vi "Text control 1 v0.2.vi"() -> ()   [LabVIEW 2016]
panel:
  in  "Panel Controls 2":T1={"Emergency Stop"=refnum, "TransGraph Max"=1e-05, "Text/Graph (text=false)"=TRUE, "TransGraph Min"=1e-11} {"TransGraph Min" format="%.2e"; "TransGraph Max" format="%.2e"}
  out "Currently running:":string="#output s 0 0 0 -0.008 0.008 0.002"
  in  "Lines left to run:":string
  in  "Standby":T2
  in  "Full Reset":bool
  in  "SMU4":cluster{"on/off":bool, "Voltage":dbl} {"Voltage" min=-100.0 max=100.0 format="%.2f"}
  in  "Source/Drain\nRange":u8(slide)=6 max=11 scale=0.0..11.0
  in  "Source/Drain\nRange mode":u16(ring) items=["Auto", "Limited", "Fixed"]
  in  "Gate Range":u8(slide)=6 max=11 scale=0.0..11.0
  in  "Gate Range\nmode":u16(ring) items=["Auto", "Limited", "Fixed"]
  in  "Gate":T3={"Gate Start"=0.0, "Gate Stop"=2.0, "Gate Step (linear only)"=1.0, "Gate Compliance"=0.0001, "Gate PComp"=0.0, "Range mode"=0, "Range"=6} {"Range" max=11 scale=0.0..11.0; "Range mode" items=["Auto", "Limited", "Fixed"]; "Gate PComp" format="%^.2e"; "Gate Compliance" format="%^.2e"; "Gate Step (linear only)" format="%^.4e"; "Gate Stop" format="%^.4e"; "Gate Start" format="%^.4e"}
  in  "Drain 2":T4={"Drain Start"=0.0, "Drain Stop"=2.0, "Drain Compliance"=0.0001, "Drain Step"=1.0, "Drain PComp"=0.0, "Range mode"=0, "Range"=6} {"Range" max=11 scale=0.0..11.0; "Range mode" items=["Auto", "Limited", "Fixed"]; "Drain PComp" format="%^.2e"; "Drain Step" format="%^.4e"; "Drain Compliance" format="%^.2e"; "Drain Stop" format="%^.4e"; "Drain Start" format="%^.4e"}
  in  "Timings 2":T5={"integration time"=0, "Short/Long integration time"=0.00064, "hold time (sec)"=0.0, "delay time (sec)"=0.0, "Step Time (0 disables)"=0.0, "sweep method"=0, "Pulse period"=0.005, "Base voltage"=0.0, "Pulse width"=0.0005} {"Pulse width" min=0.0005 max=0.1 step=0.0001 format="%.4f"; "Base voltage" format="%^.4e"; "Pulse period" min=0.005 max=1.0 step=0.0001 format="%.4f"; "sweep method" items=["Continuous", "Pulsed"]; "Step Time (0 disables)" format="%.2f"; "delay time (sec)" format="%.4f"; "hold time (sec)" format="%.4f"; "Short/Long integration time" format="%^.0e"; "integration time" scale=0.0..2.0}
  in  "Panel Controls":T6={"Emergency Stop"=refnum, "TransGraph Max"=1e-05, "Text/Graph (text=false)"=TRUE} {"TransGraph Max" format="%.2e"}
  in  "Interrupt run":bool
  in  "Drain: Compliance":dbl=0.001 format="%.8f"
  in  "Gate: Compliance":dbl=0.001 format="%.8f"
  out "Path":path=path "C:/users/rlp38/09Apr2009LTtesting/test2.txt"
  in  "hold time /s":dbl format="%.2f"
  in  "delay time /s":dbl format="%.2f"
  in  "integration time":u32(slide)=1 max=2 step=1 scale=0.0..2.0
  in  "Integration time (short)":dbl=0.0019 min=8e-05 max=0.0019 step=8e-05 format="%^.0e"
  in  "Integration time (long)":dbl=0.32 min=0.04 max=2.0 step=0.02 format="%.2f"
  in  "Step delay /s":dbl format="%.2f"
  in  "Program":string="#pulsedstressV d 0.03 20 0 0.5 0.0827 5\n#\n#itime l 0.32\n#gaterangemode a\n#drainrangemode a\n#pulsed on 0.05 0 0.02\n#transfer d -10 40 1 5 40 35\n#transfer d -10 40 1 5 40 35\n#transfer d -10 40 1 5 40 35\n#output d 0 40 20 0 40 1\n#\n#\n#sample 1 0.008 221 6 0.003\n#samplei 400e-6 200 6 0.002 0.1\n#vsu2pulse -10 4\n#\n#stressV 0.016 0.03 2e-4 0.1e-3 11\n#stressI 220e-7 0.08 15\n#transfer s -1 1 0.5 -0.005 0.005 0.005\n#output s 0 0 0 -0.008 0.008 0.002\n"
  # "Syntax:\nitime [s|m|l] time(sec): [s|m|l] determines the integration time setting (small|medium|long) and time sets the value.\nNOTE: The value of the integration time has to be within the range allowed by its category (s|m|l), otherwise, the closest value will be used. (e.g. if the category is set to short but the time value is very long, the actual value used will be the maximum short integration time.\nIntegration times:\n    Short: Default: 640 us. Range: 8E-5 - 1.92E-3 seconds.\n    Medium: Fixed at 1 NPL cycle (0.02 seconds).\n    Long: Default: 16 NPL cycles (0.32 seconds). Range: 2-100 NPL cycles (0.04 seconds - 2 seconds).\ngaterangemode [a|l|f]\ndrainrangemode [a|l|f]\npulsed [on|off] PulsePeriod(sec) PulseBaseVoltage PulseONWidth(sec)\nstandby [on l off]\nwait NumMilliseconds\nwait-min NumMinutes\n# texthere = comment\ntransfer [s|d] VgStart VgStop VgStep VdStart VdStop VdStep\noutput [s|d] VgStart VgStop VgStep VdStart VdStop VdStep\nsample Vg Vd NumSamples Time(s) SampleInterval(s)\nsamplei Idg NumSamples Time(s) SampleInterval(s) VDGcompliance\n# if in doubt use SampleInterval(s) = 0.004\nstressV VG VD IGcompliance IDcompliance Duration(sec)\nstressI IDG VDGcompliance Duration(sec)\nvsu2pulse Bias Duration(s)\npulsedstressV [s|d] VEstop VgON VgOFF Period(s) PulseONwidth(s) Vd\nsample-fpp Vg Vd NumSamples Time\nresample-fpp Vg Vd\ntransfer-fpp [s|d] VgStart VgStop VgStep VdStart VdStop VdStep\noutput-fpp [s|d] VgStart VgStop VgStep VdStart VdStop VdStep"
  # "100 samples is approx 13s with medium integration"
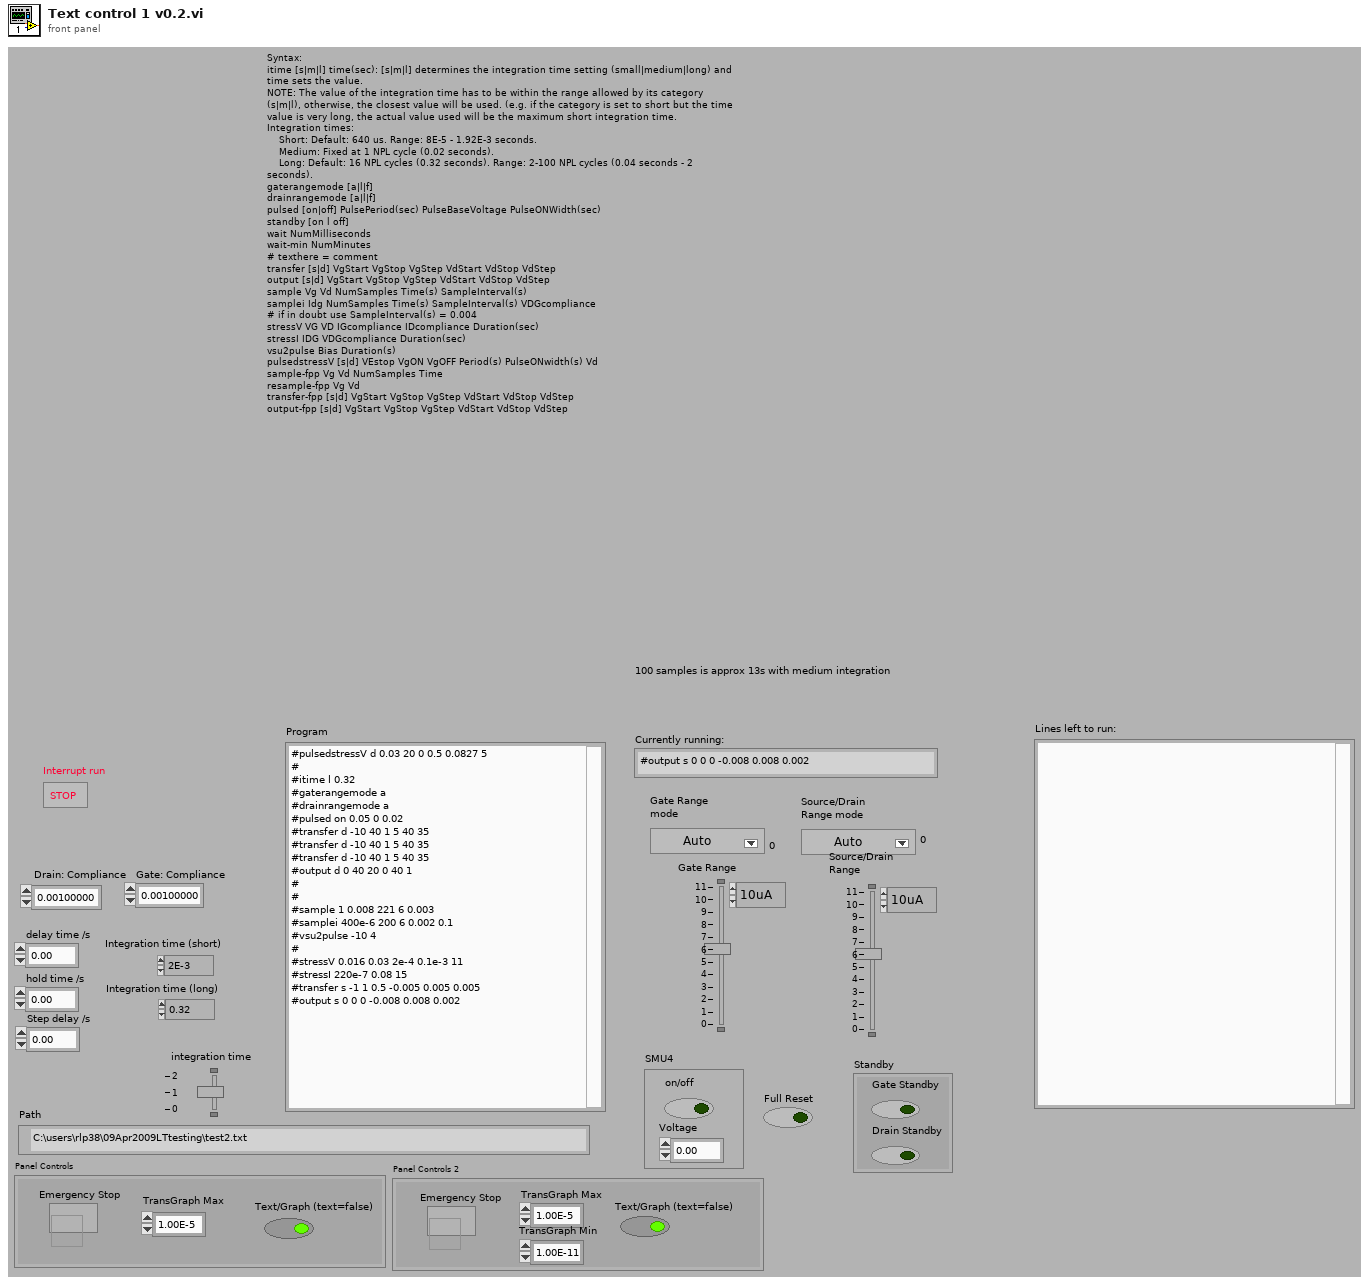
[diagram p1: front panel]
types:
  T1 = cluster{"Emergency Stop":refnum<vi>, "TransGraph Max":dbl, "Text/Graph (text=false)":bool, "TransGraph Min":dbl}
  T2 = cluster{"Gate Standby":bool, "Drain Standby":bool}
  T3 = cluster{"Gate Start":dbl, "Gate Stop":dbl, "Gate Step (linear only)":dbl, "Gate Compliance":dbl, "Gate PComp":dbl, "Range mode":u16, "Range":u8}
  T4 = cluster{"Drain Start":dbl, "Drain Stop":dbl, "Drain Compliance":dbl, "Drain Step":dbl, "Drain PComp":dbl, "Range mode":u16, "Range":u8}
  T5 = cluster{"integration time":u32, "Short/Long integration time":dbl, "hold time (sec)":dbl, "delay time (sec)":dbl, "Step Time (0 disables)":dbl, "sweep method":u16, "Pulse period":dbl, "Base voltage":dbl, "Pulse width":dbl}
  T6 = cluster{"Emergency Stop":refnum<vi>, "TransGraph Max":dbl, "Text/Graph (text=false)":bool}
  T7 = enum16{"open", "replace", "create", "open or create", "replace or create", "replace or create with confirmation"}
  T8 = cluster{"V2 Start":dbl, "V2 Step":dbl, "Number of points":i32}
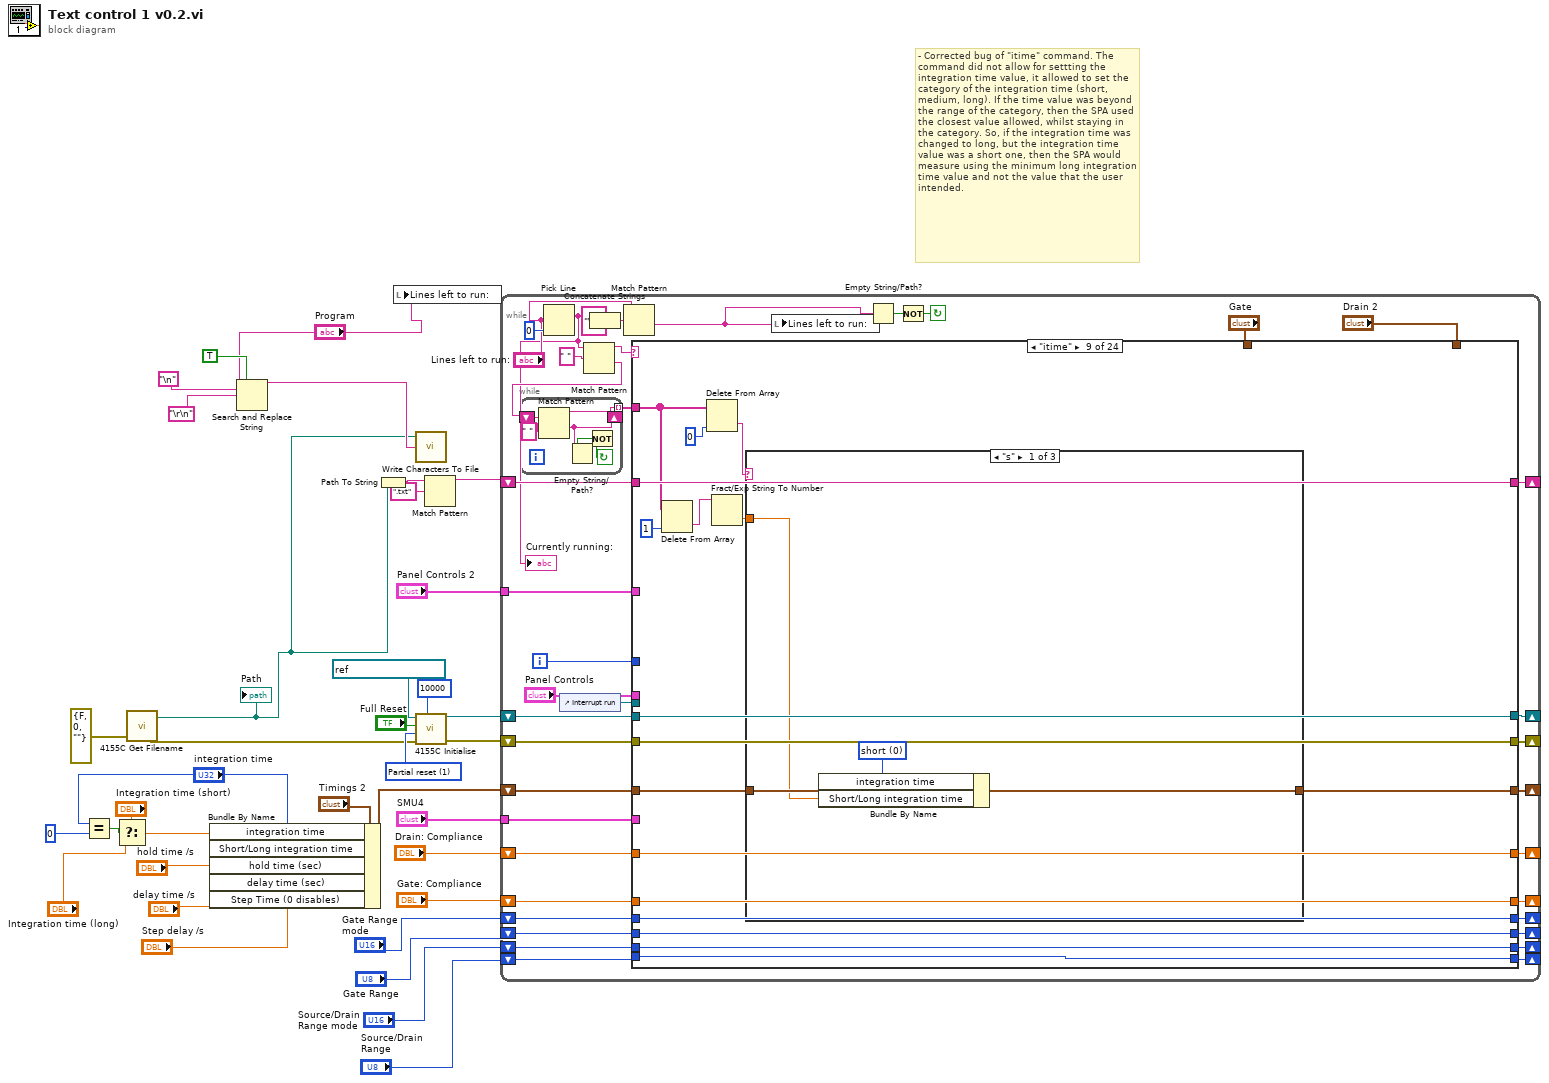
[diagram p0: block diagram]
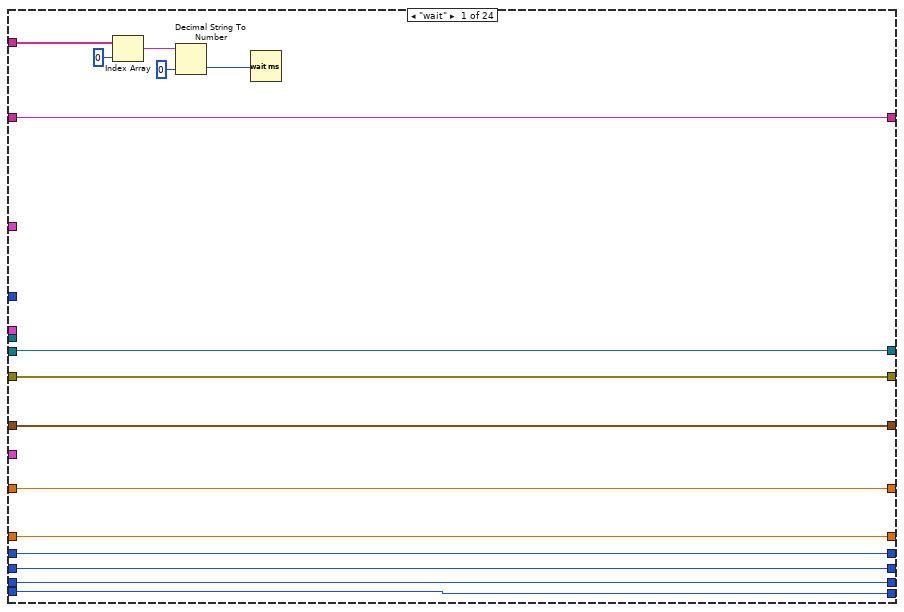
[diagram p2: hidden frame]
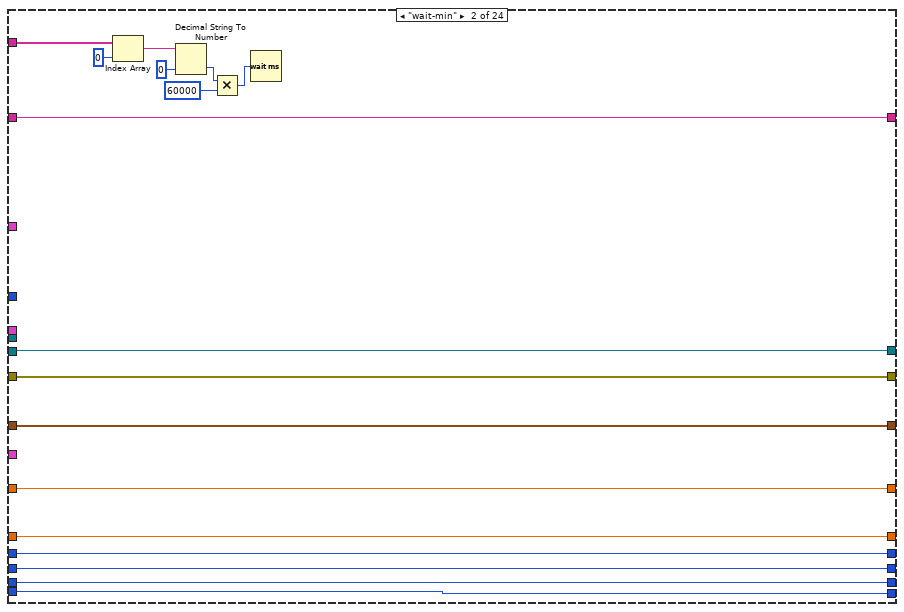
[diagram p3: hidden frame]
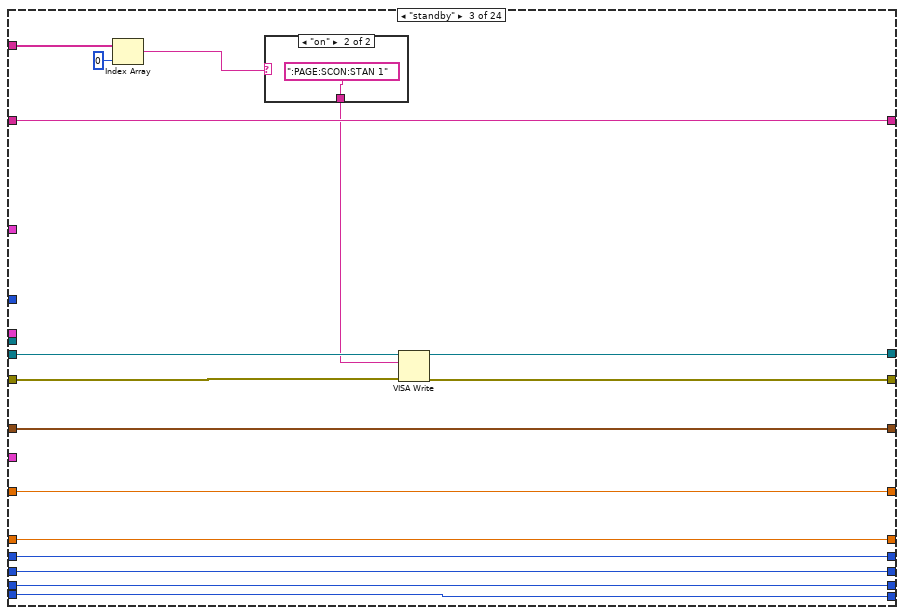
[diagram p4: hidden frame]
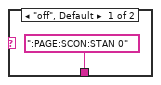
[diagram p5: hidden frame]
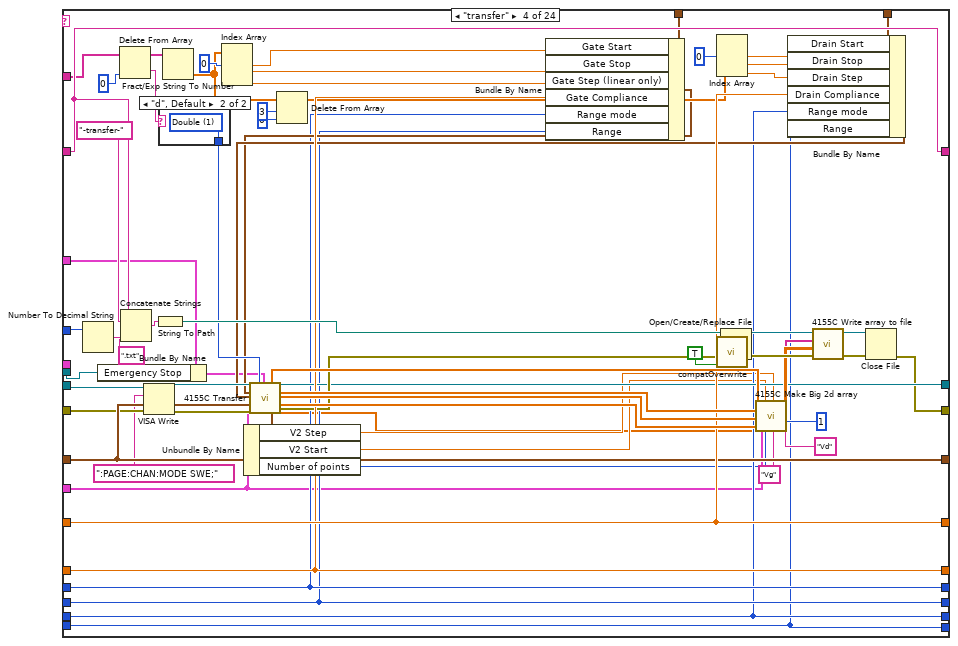
[diagram p6: hidden frame]
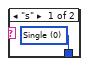
[diagram p7: hidden frame]
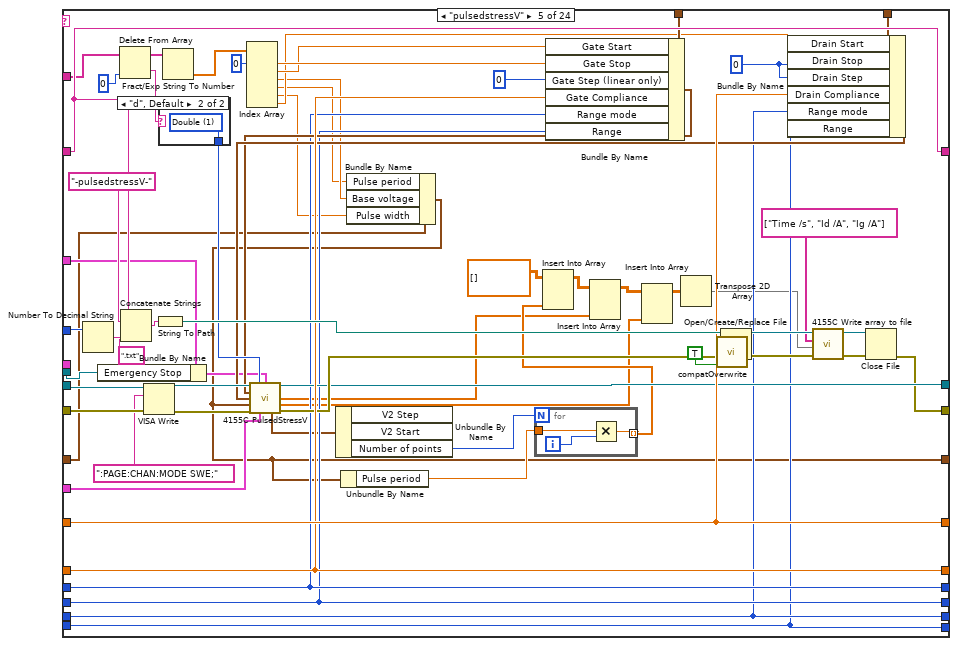
[diagram p8: hidden frame]
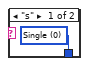
[diagram p9: hidden frame]
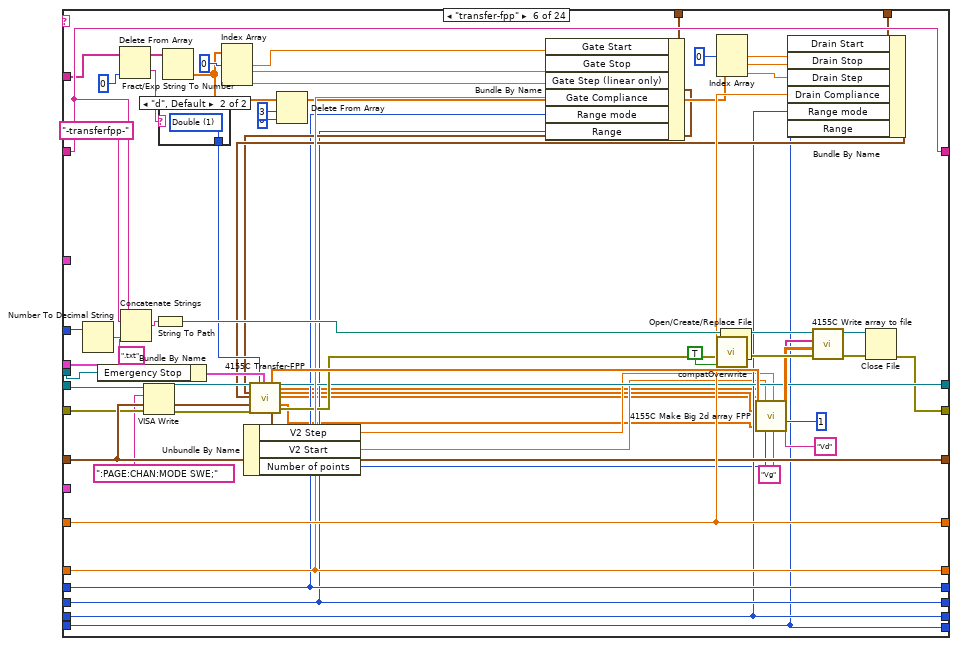
[diagram p10: hidden frame]
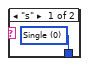
[diagram p11: hidden frame]
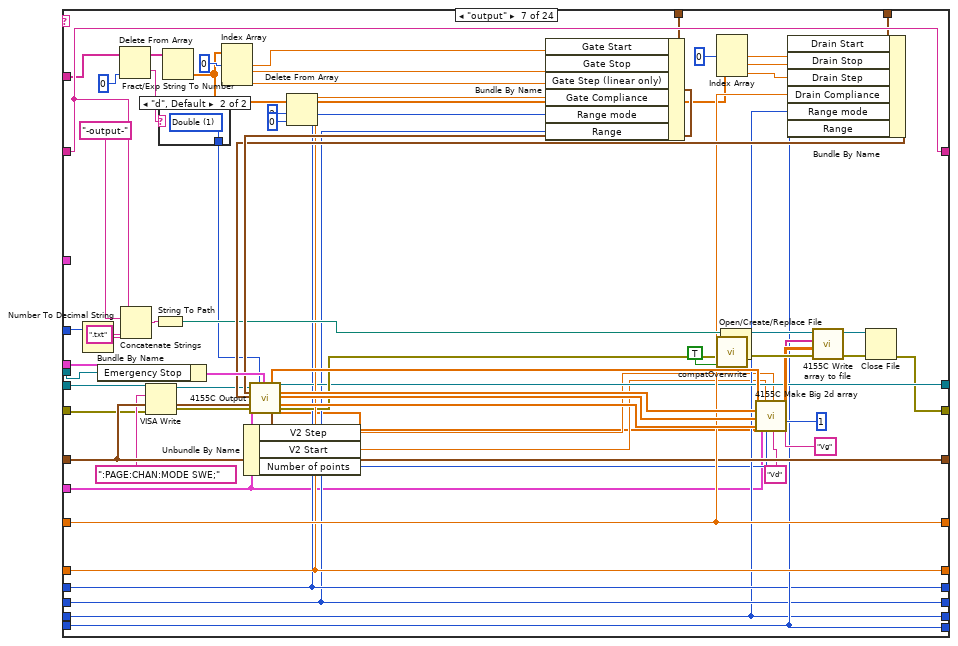
[diagram p12: hidden frame]
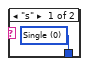
[diagram p13: hidden frame]
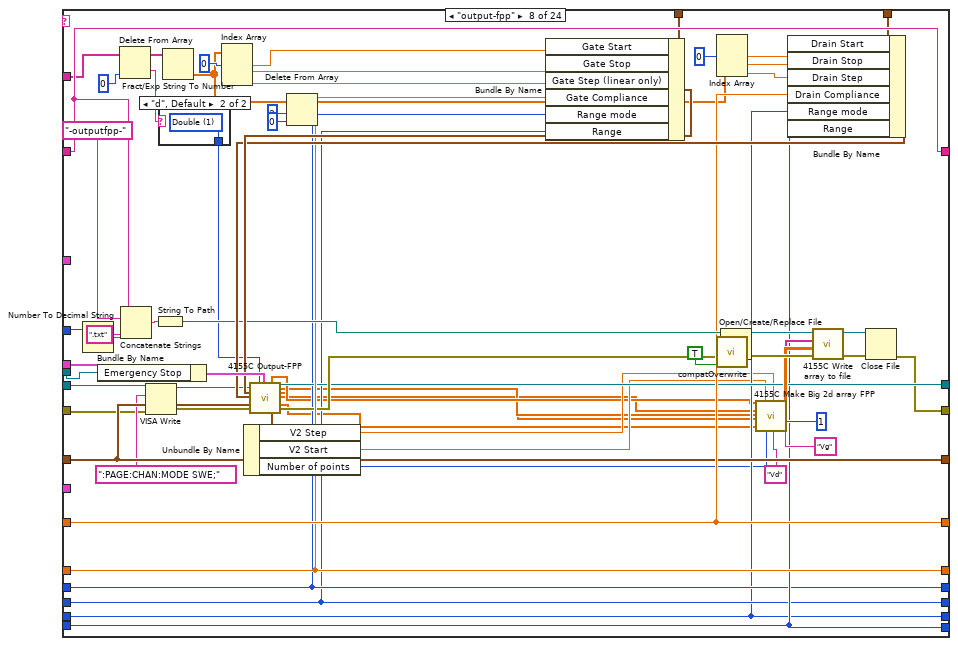
[diagram p14: hidden frame]
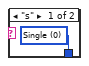
[diagram p15: hidden frame]
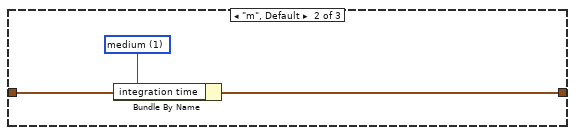
[diagram p16: hidden frame]
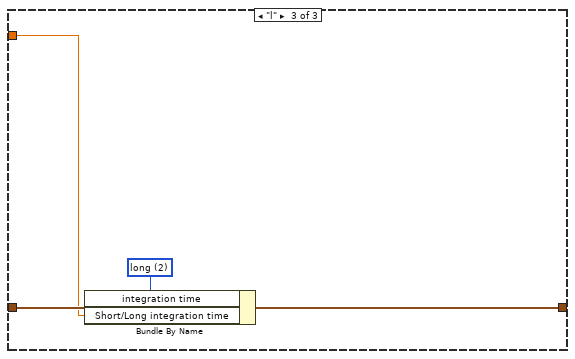
[diagram p17: hidden frame]
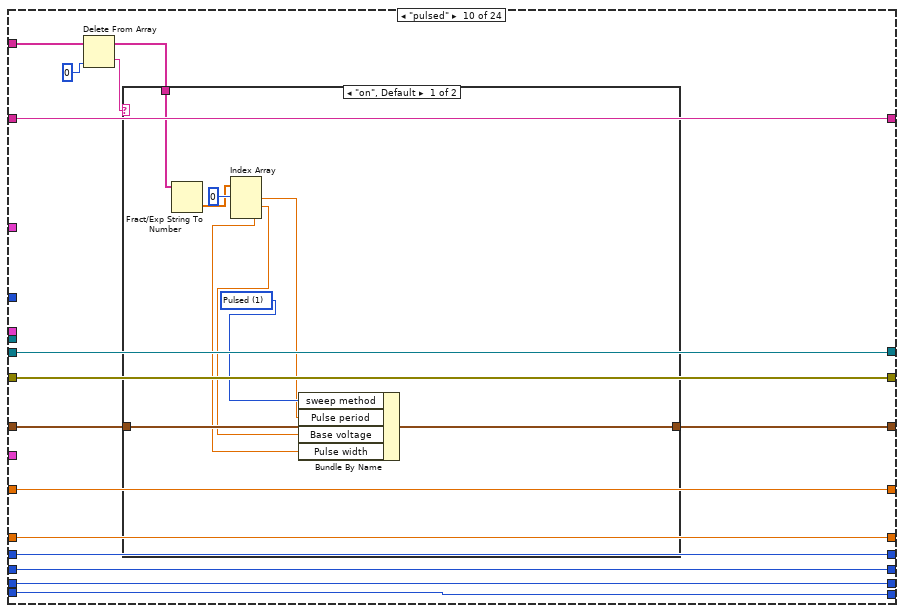
[diagram p18: hidden frame]
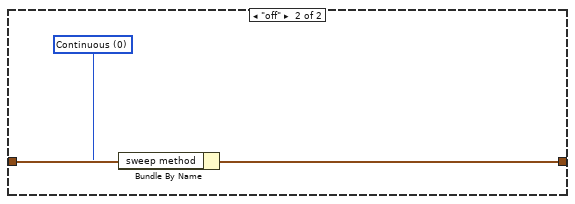
[diagram p19: hidden frame]
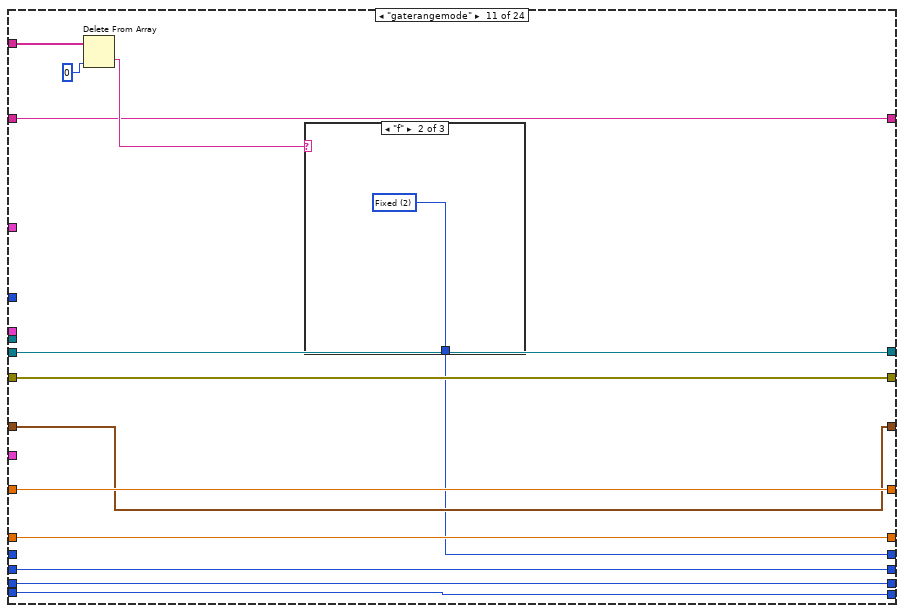
[diagram p20: hidden frame]
diagram:
  w27 = u16 1 items=["Reset All", "Partial reset"] ("Type of reset")
  # "- Corrected bug of \"itime\" command. The command did not allow for settting the integration time value, it allowed to set the category of the integration time (short, medium, long). If the time value was beyond the range of the category, then the SPA used the closest value allowed, whilst staying in the category. So, if the integration time was changed to long, but the integration time value was a short one, then the SPA would measure using the minimum long integration time value and not the value that the user intended."
  n1 = Equal?(x="integration time", y=u32 0) -> (x = y?=w31:bool)
  n2 = Select(t="Integration time (short)", s=w31, f="Integration time (long)") -> (s? t:f=w35:dbl)
  n3 = call "4155C Get Filename.vi"("error in (no error)"=errorcluster {"status"=FALSE, "code"=0, "source"=""}) -> ("error out"=w22:errorcluster, "path"=w6:path)  [unwired: 2 in, 1 out]
  "Path" <- w6
  n4 = Bundle By Name(cluster="Timings 2", "integration time"="integration time", "Short/Long integration time"=w35, "hold time (sec)"="hold time /s", "delay time (sec)"="delay time /s", "Step Time (0 disables)"="Step delay /s") -> (w19:T5)
  n5 = Search and Replace String(replace all?=TRUE ("replace all? (F)"), input string="Program", search string="\n", replace string="\r\n") -> (result string=w9:string)  [unwired: 4 in, 3 out]
  n6 = Path To String(path=w6) -> (string=w5:string)
  n7 = local write "Lines left to run:"("Program") -> ()
  n8 = call <vilib>:"Write Characters To File.vi"("character string"=w9, "file path (dialog if empty)"=w6) -> ()  [unwired: 3 in, 1 out]
  n9 = call "4155C Initialise.vi"("VISA resource name in"=refnum<visa-resource-name> "GPIB0::14::INSTR", "Reset"="Full Reset", "Type of reset"=w27, "error in (no error)"=w22, "VISA Timeout Value"=u32 10000) -> ("VISA Resource Name out"=w21:refnum<visa-resource-name>, "error out"=w20:errorcluster)
  n10 = Match Pattern(string=w5, regular expression=".txt") -> (before substring=w4:string)  [unwired: 1 in, 3 out]
  n11 = while {
    tunnel: "SMU4" -> [w41]
    shift-left: "Source/Drain\nRange" -> [w46]
    shift-right: [w42] -> _
    shift-left: "Source/Drain\nRange mode" -> [w47]
    shift-right: [w43] -> _
    shift-left: "Gate Range" -> [w48]
    shift-right: [w44] -> _
    shift-left: "Gate Range\nmode" -> [w49]
    shift-right: [w45] -> _
    shift-left: "Gate: Compliance" -> [w61]
    shift-right: [w55] -> _
    shift-left: "Drain: Compliance" -> [w62]
    shift-right: [w56] -> _
    shift-left: w19 -> [w63]
    shift-right: [w57] -> _
    shift-left: w20 -> [w64]
    shift-right: [w58] -> _
    shift-left: w21 -> [w65]
    shift-right: [w59] -> _
    shift-left: w4 -> [w66]
    shift-right: [w54] -> _
    tunnel: "Panel Controls 2" -> [w37]
    i -> [w60]
    stop <- w74 continue-if-true
    n12 = Pick Line(multi-line string="Lines left to run:", line index=0) -> (output string=w38:string)  [unwired: 1 in]
    "Currently running:" <- w38
    n13 = control-ref of="Interrupt run"() -> (w53:refnum<vi>)
    n14 = Match Pattern(string=w38, regular expression=" ") -> (before substring=w69:string, after substring=w68:string)  [unwired: 1 in, 2 out]
    n15 = while {
      tunnel: [w76] -> w67 mode=indexing
      shift-left: w68 -> [w78]
      shift-right: [w77] -> _
      stop <- w80 continue-if-true
      n16 = Match Pattern(string=w78, regular expression=" ") -> (before substring=w76:string, after substring=w77:string)  [unwired: 1 in, 2 out]
      n17 = Empty String/Path?(string/path=w77) -> (empty?=w81:bool)
      n18 = Not(x=w81) -> (.not. x?=w80:bool)
    }
    n19 = Concatenate Strings(w38, "\n" ("Substring")) -> (w72:string)
    n20 = Match Pattern(string="Lines left to run:", regular expression=w72) -> (after substring=w39:string)  [unwired: 1 in, 3 out]
    n21 = case shown="\"itime\"" w69 {
      tunnel: w67 -> [w96 w113 w129 w174 w247 w313 w377 w449 w477 w515 w540 w563 w582 w594 _ _ w689 w747 _ w807 w848 w887 w954 w1013]
      tunnel: w66 -> [w91 w109 w127 w182 w254 w321 w385 w457 w479 w504 w532 w556 w576 w587 w604 w642 w667 w729 w759 w794 w835 w875 w948 w1009]
      tunnel: w65 -> [w90 w108 w118 w152 w238 w290 w353 w425 w480 w505 w533 w557 w577 w588 w609 w645 w696 w754 w763 w814 w855 w894 w961 w966]
      tunnel: w64 -> [w89 w107 w117 w151 w237 w289 w350 w422 w481 w506 w534 w558 w578 w589 w608 w614 w695 w753 w762 w813 w854 w893 w960 w965]
      tunnel: w63 -> [w88 w106 w126 w178 w212 w317 w381 w453 w489 w514 w531 w555 w575 w586 w607 w638 w658 w721 w768 w787 w828 w868 w947 w1008]
      tunnel: w62 -> [w87 w105 w125 w180 w252 w319 w383 w455 w488 w513 w539 w562 w581 w593 w606 w623 w694 w752 w771 w812 w853 w892 w959 w1018]
      tunnel: w61 -> [w86 w104 w124 w179 w251 w318 w382 w454 w487 w512 w538 w561 w580 w592 w605 w624 w668 w730 w770 w795 w836 w876 w949 w1010]
      tunnel: w60 -> [_ _ _ w183 w255 w322 w386 w458 _ _ _ _ _ _ _ w640 w693 w751 _ w811 w852 w891 w958 w1017]
      tunnel: [w90 w108 w116 w176 w249 w315 w379 w451 w480 w505 w533 w557 w577 w588 w609 w645 w659 w702 w761 w788 w829 w869 w899 w968] -> w59
      tunnel: [w89 w107 w115 w175 w248 w314 w378 w450 w481 w506 w534 w558 w578 w589 w608 w613 w669 w703 w760 w796 w837 w877 w898 w967] -> w58
      tunnel: [w88 w106 w126 w178 w208 w317 w381 w453 w482 w507 w531 w555 w575 w586 w607 w638 w658 w721 w768 w787 w828 w868 w947 w1008] -> w57
      tunnel: [w87 w105 w125 w180 w252 w319 w383 w455 w488 w513 w539 w562 w581 w593 w606 w623 w694 w752 w771 w812 w853 w892 w959 w1018] -> w56
      tunnel: [w86 w104 w124 w179 w251 w318 w382 w454 w487 w512 w538 w561 w580 w592 w605 w624 w668 w730 w770 w795 w836 w876 w949 w1010] -> w55
      tunnel: [w91 w109 w127 w182 w254 w321 w385 w457 w479 w504 w532 w556 w576 w587 w604 w642 w667 w729 w759 w794 w835 w875 w948 w1009] -> w54
      tunnel: w53 -> [_ _ _ w191 w259 w327 w394 w462 _ _ _ _ _ _ _ _ w664 w726 _ w793 w834 w874 w919 w984]
      tunnel: "Gate" -> [_ _ _ w161 w241 w300 w364 w436 _ _ _ _ _ _ _ _ _ _ _ _ _ _ _ _]
      tunnel: "Drain 2" -> [_ _ _ w160 w240 w299 w363 w435 _ _ _ _ _ _ _ _ _ _ _ _ _ _ _ _]
      tunnel: "Panel Controls" -> [_ _ _ _ _ w298 w362 w434 _ _ _ _ _ _ _ _ _ _ _ _ _ _ _ _]
      tunnel: w49 -> [w85 w103 w123 w145 w231 w283 w348 w420 w486 w511 _ w554 w574 w585 w603 w625 w654 w717 w764 w783 w824 w864 w943 w1004]
      tunnel: w48 -> [w84 w102 w122 w144 w230 w282 w347 w419 w485 w510 w537 _ w565 w591 w602 w626 w655 w718 w765 w784 w825 w865 w944 w1005]
      tunnel: w47 -> [w83 w101 w121 w143 w229 w281 w346 w418 w484 w509 w536 w560 w579 _ w601 w627 w656 w719 w766 w785 w826 w866 w945 w1006]
      tunnel: w46 -> [w82 w100 w120 w142 w228 w280 w349 w421 w483 w508 w535 w559 _ w590 w600 w628 w657 w720 w767 w786 w827 w867 w946 w1007]
      tunnel: [w85 w103 w123 w145 w231 w283 w348 w420 w486 w511 w530 w554 w574 w585 w603 w625 w654 w717 w764 w783 w824 w864 w943 w1004] -> w45
      tunnel: [w84 w102 w122 w144 w230 w282 w347 w419 w485 w510 w537 w546 w565 w591 w602 w626 w655 w718 w765 w784 w825 w865 w944 w1005] -> w44
      tunnel: [w83 w101 w121 w143 w229 w281 w346 w418 w484 w509 w536 w560 w579 w584 w601 w627 w656 w719 w766 w785 w826 w866 w945 w1006] -> w43
      tunnel: [w82 w100 w120 w142 w228 w280 w349 w421 w483 w508 w535 w559 w566 w590 w600 w628 w657 w720 w767 w786 w827 w867 w946 w1007] -> w42
      tunnel: w41 -> [_ _ _ w135 w224 _ w340 _ _ _ _ _ _ _ _ _ _ _ _ _ _ _ _ _]
      tunnel: w37 -> [_ _ _ w133 w223 _ _ _ _ _ _ _ _ _ _ _ _ _ _ _ _ _ _ _]
      frame "wait" {
        n22 = Index Array(array=w96, index=0 ("Index")) -> (element=w94:string)
        n23 = Decimal String To Number(string=w94, default (0L)=u32 0) -> (number=w93:u32)  [unwired: 1 in, 1 out]
        n24 = Wait (ms)(milliseconds to wait=w93) -> ()  [unwired: 1 out]
      }
      frame "wait-min" {
        n25 = Index Array(array=w113, index=0 ("Index")) -> (element=w111:string)
        n26 = Decimal String To Number(string=w111, default (0L)=u32 0) -> (number=w99:u32)  [unwired: 1 in, 1 out]
        n27 = Multiply(x=w99, y=u32 60000) -> (x*y=w98:u32)
        n28 = Wait (ms)(milliseconds to wait=w98) -> ()  [unwired: 1 out]
      }
      frame "standby" {
        n29 = Index Array(array=w129, index=0 ("Index")) -> (element=w119:string)
        n30 = case shown="\"on\"" w119 {
          tunnel: [":PAGE:SCON:STAN 0" ":PAGE:SCON:STAN 1"] -> w114
          frame "off", Default {
          }
          frame "on" {
          }
        }
        n31 = VISA Write(VISA resource name=w118, write buffer=w114, error in (no error)=w117) -> (VISA resource name out=w116:refnum<visa-resource-name>, error out=w115:errorcluster)  [unwired: 1 out]
      }
      frame "transfer" {
        n32 = Number To Decimal String(number=w183) -> (decimal integer string=w184:string)  [unwired: 1 in]
        n33 = Bundle By Name(cluster=w133, "Emergency Stop"=w191) -> (w134:T1)
        n34 = Delete From Array(array=w174, index=0 ("Index")) -> (deleted portion=w172:string, array with subset deleted=w171:string[])  [unwired: 1 in]
        n35 = Concatenate Strings(w182, "-transfer-" ("Substring"), w184, ".txt" ("Substring")) -> (w186:string)
        n36 = VISA Write(VISA resource name=w152, write buffer=":PAGE:CHAN:MODE SWE;" ("write buffer (\"\")"), error in (no error)=w151) -> (VISA resource name out=w149:refnum<visa-resource-name>, error out=w150:errorcluster)  [unwired: 1 out]
        n37 = String To Path(string=w186) -> (path=w181:path)
        n38 = case shown="\"d\", Default" w172 {
          tunnel: [w199 w200] -> w170
          frame "s" {
            w199 = u16 0 items=["Single", "Double"] ("sweep mode")
          }
          frame "d", Default {
            w200 = u16 1 items=["Single", "Double"] ("sweep mode")
          }
        }
        n39 = Fract/Exp String To Number(string=w171) -> (number=w156:dbl[])  [unwired: 3 in, 1 out]
        n40 = Index Array(array=w156, index #1=0 ("Index")) -> (element #1=w169:dbl, element #2=w168:dbl, element #3=w167:dbl)  [unwired: 2 in]
        n41 = Delete From Array(array=w156, length=3 ("Length"), index=0 ("Index")) -> (array with subset deleted=w154:dbl[])  [unwired: 1 out]
        n42 = Bundle By Name(cluster=w161, "Gate Start"=w169, "Gate Stop"=w168, "Gate Step (linear only)"=w167, "Gate Compliance"=w179, "Range mode"=w145, "Range"=w144) -> (w146:T3)
        n43 = Index Array(array=w154, index #1=0 ("Index")) -> (element #1=w164:dbl, element #2=w163:dbl, element #3=w162:dbl)  [unwired: 2 in]
        n44 = call <vilib>:"compatOverwrite.vi"("overwrite (F)"=TRUE) -> ("overwrite?"=w132:T7)
        n45 = Bundle By Name(cluster=w160, "Drain Start"=w164, "Drain Stop"=w163, "Drain Step"=w162, "Drain Compliance"=w180, "Range mode"=w143, "Range"=w142) -> (w147:T4)
        n46 = call "4155C Transfer.vi"("VISA resource name in"=w149, "Gate"=w146, "Drain"=w147, "Timings"=w178, "error in (no error)"=w150, "SMU4"=w135, "sweep mode"=w170, "Panel Controls"=w134) -> ("VG"=w187:dbl[], "Outparams"=w140:T8, "VISA Resource Name out"=w176:refnum<visa-resource-name>, "IS"=w190:dbl[], "ID"=w189:dbl[], "IG"=w188:dbl[], "error out"=w177:errorcluster, "SMU4"=w136:dbl[])  [unwired: 12 in]
        n47 = Unbundle By Name(w140) -> ("V2 Step"=w139:dbl, "V2 Start"=w138:dbl, "Number of points"=w137:i32)
        n48 = Open/Create/Replace File(file path (use dialog)=w181, error in=w177, operation (0:open)=w132) -> (refnum out=w196:refnum<file>, error out=w197:errorcluster)  [unwired: 3 in, 1 out]
        n49 = call "4155C Make Big 2d array.vi"("1D Var1"=w187, "1d IS"=w190, "1d ID"=w189, "1d IG"=w188, "1d SMU4"=w136, "SMU4"=w135, "VAR2 START"=w138, "Number of VAR2 steps"=w137, "VAR2 STEP"=w139, "VAR1 Name"="Vg", "Decimal places in header"=i8 1, "VAR2 Name"="Vd") -> ("Header array"=w192:string[], "Data array"=w193:dbl[][])  [unwired: 14 in]
        n50 = call "4155C Write array to file.vi"("Byte Stream File Refnum"=w196, "Header"=w192, "Data Array"=w193, "error in (no error)"=w197) -> ("dup refnum"=w194:refnum<file>, "error out"=w195:errorcluster)  [unwired: 1 in]
        n51 = Close File(refnum=w194, error in=w195) -> (error out=w175:errorcluster)  [unwired: 1 out]
      }
      frame "pulsedstressV" {
        w206 = 0
        n52 = Number To Decimal String(number=w255) -> (decimal integer string=w256:string)  [unwired: 1 in]
        n53 = Bundle By Name(cluster=w223, "Emergency Stop"=w259) -> (w225:T1)
        n54 = Delete From Array(array=w247, index=0 ("Index")) -> (deleted portion=w245:string, array with subset deleted=w244:string[])  [unwired: 1 in]
        n55 = Concatenate Strings(w254, "-pulsedstressV-" ("Substring"), w256, ".txt" ("Substring")) -> (w258:string)
        n56 = VISA Write(VISA resource name=w238, write buffer=":PAGE:CHAN:MODE SWE;" ("write buffer (\"\")"), error in (no error)=w237) -> (VISA resource name out=w235:refnum<visa-resource-name>, error out=w236:errorcluster)  [unwired: 1 out]
        n57 = String To Path(string=w258) -> (path=w253:path)
        n58 = case shown="\"d\", Default" w245 {
          tunnel: [w268 w269] -> w243
          frame "s" {
            w268 = u16 0 items=["Single", "Double"] ("sweep mode")
          }
          frame "d", Default {
            w269 = u16 1 items=["Single", "Double"] ("sweep mode")
          }
        }
        n59 = Fract/Exp String To Number(string=w244) -> (number=w239:dbl[])  [unwired: 3 in, 1 out]
        n60 = Index Array(array=w239, index #1=0 ("Index")) -> (element #1=w215:dbl, element #2=w214:dbl, element #3=w211:dbl, element #4=w210:dbl, element #5=w209:dbl, element #6=w213:dbl)  [unwired: 5 in]
        n61 = Bundle By Name(cluster=w212, "Pulse period"=w210, "Base voltage"=w211, "Pulse width"=w209) -> (w208:T5)
        n62 = Unbundle By Name(w208) -> ("Pulse period"=w216:dbl)
        n63 = Bundle By Name(cluster=w241, "Gate Start"=w214, "Gate Stop"=w215, "Gate Step (linear only)"=0, "Gate Compliance"=w251, "Range mode"=w231, "Range"=w230) -> (w232:T3)
        n64 = call <vilib>:"compatOverwrite.vi"("overwrite (F)"=TRUE) -> ("overwrite?"=w201:T7)
        n65 = Bundle By Name(cluster=w240, "Drain Start"=w213, "Drain Stop"=w206, "Drain Step"=w206, "Drain Compliance"=w252, "Range mode"=w229, "Range"=w228) -> (w233:T4)
        n66 = call "4155C PulsedStressV.vi"("VISA resource name in"=w235, "sweep mode"=w243, "Panel Controls"=w225, "Gate"=w232, "Drain"=w233, "Timings"=w208, "error in (no error)"=w236, "SMU4"=w224) -> ("VISA Resource Name out"=w249:refnum<visa-resource-name>, "ID"=w204:dbl[], "IG"=w202:dbl[], "Outparams"=w226:T8, "error out"=w250:errorcluster)  [unwired: 3 in]
        n67 = Unbundle By Name(w226) -> ("Number of points"=w203:i32)  [unwired: 2 out]
        n68 = for {
          N: w203 -> [_]
          tunnel: [w265] -> w205 mode=indexing
          tunnel: w216 -> [w267]
          i -> [w266]
          n69 = Multiply(x=w267, y=w266) -> (x*y=w265:dbl)
        }
        n70 = Insert Into Array(array=dbl[][] [] ("Input Array"), new element=w205) -> (w217:dbl[][])  [unwired: 2 in]
        n71 = Insert Into Array(array=w217, new element=w204) -> (w222:dbl[][])  [unwired: 2 in]
        n72 = Insert Into Array(array=w222, new element=w202) -> (w221:dbl[][])  [unwired: 2 in]
        n73 = Transpose 2D Array(2D array=w221) -> (transposed array=w220:dbl[][])
        n74 = Open/Create/Replace File(file path (use dialog)=w253, error in=w250, operation (0:open)=w201) -> (refnum out=w262:refnum<file>, error out=w263:errorcluster)  [unwired: 3 in, 1 out]
        n75 = call "4155C Write array to file.vi"("Byte Stream File Refnum"=w262, "Header"=string[] ["Time /s", "Id /A", "Ig /A"], "Data Array"=w220, "error in (no error)"=w263) -> ("dup refnum"=w260:refnum<file>, "error out"=w261:errorcluster)  [unwired: 1 in]
        n76 = Close File(refnum=w260, error in=w261) -> (error out=w248:errorcluster)  [unwired: 1 out]
      }
      frame "transfer-fpp" {
        n77 = Number To Decimal String(number=w322) -> (decimal integer string=w323:string)  [unwired: 1 in]
        n78 = Bundle By Name(cluster=w298, "Emergency Stop"=w327) -> (w335:T6)
        n79 = Delete From Array(array=w313, index=0 ("Index")) -> (deleted portion=w311:string, array with subset deleted=w310:string[])  [unwired: 1 in]
        n80 = Concatenate Strings(w321, "-transferfpp-" ("Substring"), w323, ".txt" ("Substring")) -> (w325:string)
        n81 = VISA Write(VISA resource name=w290, write buffer=":PAGE:CHAN:MODE SWE;" ("write buffer (\"\")"), error in (no error)=w289) -> (VISA resource name out=w287:refnum<visa-resource-name>, error out=w288:errorcluster)  [unwired: 1 out]
        n82 = String To Path(string=w325) -> (path=w320:path)
        n83 = case shown="\"d\", Default" w311 {
          tunnel: [w336 w337] -> w309
          frame "s" {
            w336 = u16 0 items=["Single", "Double"] ("sweep mode")
          }
          frame "d", Default {
            w337 = u16 1 items=["Single", "Double"] ("sweep mode")
          }
        }
        n84 = Fract/Exp String To Number(string=w310) -> (number=w294:dbl[])  [unwired: 3 in, 1 out]
        n85 = Index Array(array=w294, index #1=0 ("Index")) -> (element #1=w308:dbl, element #2=w307:dbl, element #3=w306:dbl)  [unwired: 2 in]
        n86 = Delete From Array(array=w294, length=3 ("Length"), index=0 ("Index")) -> (array with subset deleted=w292:dbl[])  [unwired: 1 out]
        n87 = Bundle By Name(cluster=w300, "Gate Start"=w308, "Gate Stop"=w307, "Gate Step (linear only)"=w306, "Gate Compliance"=w318, "Range mode"=w283, "Range"=w282) -> (w284:T3)
        n88 = Index Array(array=w292, index #1=0 ("Index")) -> (element #1=w303:dbl, element #2=w302:dbl, element #3=w301:dbl)  [unwired: 2 in]
        n89 = call <vilib>:"compatOverwrite.vi"("overwrite (F)"=TRUE) -> ("overwrite?"=w270:T7)
        n90 = Bundle By Name(cluster=w299, "Drain Start"=w303, "Drain Stop"=w302, "Drain Step"=w301, "Drain Compliance"=w319, "Range mode"=w281, "Range"=w280) -> (w285:T4)
        n91 = call "4155C Transfer-FPP.vi"("VISA resource name in"=w287, "Gate"=w284, "Drain"=w285, "Timings"=w317, "error in (no error)"=w288, "sweep mode"=w309, "Panel Controls"=w335) -> ("VG"=w326:dbl[], "Outparams"=w278:T8, "VISA Resource Name out"=w315:refnum<visa-resource-name>, "Vprobe2"=w274:dbl[], "ID"=w273:dbl[], "IG"=w272:dbl[], "Vprobe1"=w271:dbl[], "error out"=w316:errorcluster)  [unwired: 13 in]
        n92 = Unbundle By Name(w278) -> ("V2 Step"=w277:dbl, "V2 Start"=w276:dbl, "Number of points"=w275:i32)
        n93 = Open/Create/Replace File(file path (use dialog)=w320, error in=w316, operation (0:open)=w270) -> (refnum out=w332:refnum<file>, error out=w333:errorcluster)  [unwired: 3 in, 1 out]
        n94 = call "4155C Make Big 2d array FPP.vi"("1D Var1"=w326, "1d ID"=w273, "1d Vp2"=w274, "1d IG"=w272, "1d Vp1"=w271, "VAR2 START"=w276, "Number of VAR2 steps"=w275, "VAR2 STEP"=w277, "VAR1 Name"="Vg", "Decimal places in header"=i8 1, "VAR2 Name"="Vd") -> ("Header array"=w328:string[], "Data array"=w329:dbl[][])  [unwired: 15 in]
        n95 = call "4155C Write array to file.vi"("Byte Stream File Refnum"=w332, "Header"=w328, "Data Array"=w329, "error in (no error)"=w333) -> ("dup refnum"=w330:refnum<file>, "error out"=w331:errorcluster)  [unwired: 1 in]
        n96 = Close File(refnum=w330, error in=w331) -> (error out=w314:errorcluster)  [unwired: 1 out]
      }
      frame "output" {
        n97 = Number To Decimal String(number=w386) -> (decimal integer string=w387:string)  [unwired: 1 in]
        n98 = Bundle By Name(cluster=w362, "Emergency Stop"=w394) -> (w404:T6)
        n99 = Delete From Array(array=w377, index=0 ("Index")) -> (deleted portion=w375:string, array with subset deleted=w374:string[])  [unwired: 1 in]
        n100 = Concatenate Strings(w385, "-output-" ("Substring"), w387, ".txt" ("Substring")) -> (w389:string)
        n101 = VISA Write(VISA resource name=w353, write buffer=":PAGE:CHAN:MODE SWE;" ("write buffer (\"\")"), error in (no error)=w350) -> (VISA resource name out=w352:refnum<visa-resource-name>, error out=w351:errorcluster)  [unwired: 1 out]
        n102 = String To Path(string=w389) -> (path=w384:path)
        n103 = case shown="\"d\", Default" w375 {
          tunnel: [w405 w406] -> w373
          frame "s" {
            w405 = u16 0 items=["Single", "Double"] ("sweep mode")
          }
          frame "d", Default {
            w406 = u16 1 items=["Single", "Double"] ("sweep mode")
          }
        }
        n104 = Fract/Exp String To Number(string=w374) -> (number=w356:dbl[])  [unwired: 3 in, 1 out]
        n105 = Index Array(array=w356, index #1=0 ("Index")) -> (element #1=w372:dbl, element #2=w371:dbl, element #3=w370:dbl)  [unwired: 2 in]
        n106 = Delete From Array(array=w356, length=3 ("Length"), index=0 ("Index")) -> (array with subset deleted=w355:dbl[])  [unwired: 1 out]
        n107 = Bundle By Name(cluster=w364, "Gate Start"=w372, "Gate Stop"=w371, "Gate Step (linear only)"=w370, "Gate Compliance"=w382, "Range mode"=w348, "Range"=w347) -> (w403:T3)
        n108 = Index Array(array=w355, index #1=0 ("Index")) -> (element #1=w367:dbl, element #2=w366:dbl, element #3=w365:dbl)  [unwired: 2 in]
        n109 = call <vilib>:"compatOverwrite.vi"("overwrite (F)"=TRUE) -> ("overwrite?"=w338:T7)
        n110 = Bundle By Name(cluster=w363, "Drain Start"=w367, "Drain Stop"=w366, "Drain Step"=w365, "Drain Compliance"=w383, "Range mode"=w346, "Range"=w349) -> (w402:T4)
        n111 = call "4155C Output.vi"("VISA resource name in"=w352, "Gate"=w403, "Drain"=w402, "Timings"=w381, "error in (no error)"=w351, "SMU4"=w340, "sweep mode"=w373, "Panel controls"=w404) -> ("VD"=w390:dbl[], "Outparams"=w343:T8, "VISA Resource Name out"=w379:refnum<visa-resource-name>, "IS"=w393:dbl[], "ID"=w392:dbl[], "IG"=w391:dbl[], "error out"=w380:errorcluster, "SMU4"=w339:dbl[])  [unwired: 12 in]
        n112 = Unbundle By Name(w343) -> ("V2 Step"=w344:dbl, "V2 Start"=w342:dbl, "Number of points"=w341:i32)
        n113 = Open/Create/Replace File(file path (use dialog)=w384, error in=w380, operation (0:open)=w338) -> (refnum out=w399:refnum<file>, error out=w400:errorcluster)  [unwired: 3 in, 1 out]
        n114 = call "4155C Make Big 2d array.vi"("1D Var1"=w390, "1d IS"=w393, "1d ID"=w392, "1d IG"=w391, "1d SMU4"=w339, "SMU4"=w340, "VAR2 START"=w342, "Number of VAR2 steps"=w341, "VAR2 STEP"=w344, "VAR1 Name"="Vd", "Decimal places in header"=i8 1, "VAR2 Name"="Vg") -> ("Header array"=w395:string[], "Data array"=w396:dbl[][])  [unwired: 14 in]
        n115 = call "4155C Write array to file.vi"("Byte Stream File Refnum"=w399, "Header"=w395, "Data Array"=w396, "error in (no error)"=w400) -> ("dup refnum"=w397:refnum<file>, "error out"=w398:errorcluster)  [unwired: 1 in]
        n116 = Close File(refnum=w397, error in=w398) -> (error out=w378:errorcluster)  [unwired: 1 out]
      }
      frame "output-fpp" {
        n117 = Number To Decimal String(number=w458) -> (decimal integer string=w459:string)  [unwired: 1 in]
        n118 = Bundle By Name(cluster=w434, "Emergency Stop"=w462) -> (w472:T6)
        n119 = Delete From Array(array=w449, index=0 ("Index")) -> (deleted portion=w447:string, array with subset deleted=w446:string[])  [unwired: 1 in]
        n120 = Concatenate Strings(w457, "-outputfpp-" ("Substring"), w459, ".txt" ("Substring")) -> (w461:string)
        n121 = VISA Write(VISA resource name=w425, write buffer=":PAGE:CHAN:MODE SWE;" ("write buffer (\"\")"), error in (no error)=w422) -> (VISA resource name out=w424:refnum<visa-resource-name>, error out=w423:errorcluster)  [unwired: 1 out]
        n122 = String To Path(string=w461) -> (path=w456:path)
        n123 = case shown="\"d\", Default" w447 {
          tunnel: [w473 w474] -> w445
          frame "s" {
            w473 = u16 0 items=["Single", "Double"] ("sweep mode")
          }
          frame "d", Default {
            w474 = u16 1 items=["Single", "Double"] ("sweep mode")
          }
        }
        n124 = Fract/Exp String To Number(string=w446) -> (number=w428:dbl[])  [unwired: 3 in, 1 out]
        n125 = Index Array(array=w428, index #1=0 ("Index")) -> (element #1=w444:dbl, element #2=w443:dbl, element #3=w442:dbl)  [unwired: 2 in]
        n126 = Delete From Array(array=w428, length=3 ("Length"), index=0 ("Index")) -> (array with subset deleted=w427:dbl[])  [unwired: 1 out]
        n127 = Bundle By Name(cluster=w436, "Gate Start"=w444, "Gate Stop"=w443, "Gate Step (linear only)"=w442, "Gate Compliance"=w454, "Range mode"=w420, "Range"=w419) -> (w471:T3)
        n128 = Index Array(array=w427, index #1=0 ("Index")) -> (element #1=w439:dbl, element #2=w438:dbl, element #3=w437:dbl)  [unwired: 2 in]
        n129 = call <vilib>:"compatOverwrite.vi"("overwrite (F)"=TRUE) -> ("overwrite?"=w407:T7)
        n130 = Bundle By Name(cluster=w435, "Drain Start"=w439, "Drain Stop"=w438, "Drain Step"=w437, "Drain Compliance"=w455, "Range mode"=w418, "Range"=w421) -> (w470:T4)
        n131 = call "4155C Output-FPP.vi"("VISA resource name in"=w424, "Gate"=w471, "Drain"=w470, "Timings"=w453, "error in (no error)"=w423, "sweep mode"=w445, "Panel controls"=w472) -> ("VD"=w412:dbl[], "Outparams"=w415:T8, "VISA Resource Name out"=w451:refnum<visa-resource-name>, "Vprobe2"=w411:dbl[], "ID"=w410:dbl[], "IG"=w409:dbl[], "Vprobe1"=w408:dbl[], "error out"=w452:errorcluster)  [unwired: 13 in]
        n132 = Unbundle By Name(w415) -> ("V2 Step"=w416:dbl, "V2 Start"=w414:dbl, "Number of points"=w413:i32)
        n133 = Open/Create/Replace File(file path (use dialog)=w456, error in=w452, operation (0:open)=w407) -> (refnum out=w467:refnum<file>, error out=w468:errorcluster)  [unwired: 3 in, 1 out]
        n134 = call "4155C Make Big 2d array FPP.vi"("1D Var1"=w412, "1d ID"=w410, "1d Vp2"=w411, "1d IG"=w409, "1d Vp1"=w408, "VAR2 START"=w414, "Number of VAR2 steps"=w413, "VAR2 STEP"=w416, "VAR1 Name"="Vd", "Decimal places in header"=i8 1, "VAR2 Name"="Vg") -> ("Header array"=w463:string[], "Data array"=w464:dbl[][])  [unwired: 15 in]
        n135 = call "4155C Write array to file.vi"("Byte Stream File Refnum"=w467, "Header"=w463, "Data Array"=w464, "error in (no error)"=w468) -> ("dup refnum"=w465:refnum<file>, "error out"=w466:errorcluster)  [unwired: 1 in]
        n136 = Close File(refnum=w465, error in=w466) -> (error out=w450:errorcluster)  [unwired: 1 out]
      }
      frame "itime" {
        n137 = Delete From Array(array=w477, index=1) -> (deleted portion=w476:string)  [unwired: 1 in, 1 out]
        n138 = Delete From Array(array=w477, index=0 ("Index")) -> (deleted portion=w490:string)  [unwired: 1 in, 1 out]
        n139 = Fract/Exp String To Number(string=w476) -> (number=w475:dbl)  [unwired: 3 in, 1 out]
        n140 = case shown="\"s\"" w490 {
          tunnel: w489 -> [w495 w497 w501]
          tunnel: [w494 w496 w500] -> w482
          tunnel: w475 -> [w492 _ w499]
          frame "s" {
            w493 = u32 0 items=["short  ", "medium  ", "long  "] ("integration time 2")
            n141 = Bundle By Name(cluster=w495, "integration time"=w493, "Short/Long integration time"=w492) -> (w494:T5)
          }
          frame "m", Default {
            w498 = u32 1 items=["short  ", "medium  ", "long  "] ("integration time 2")
            n142 = Bundle By Name(cluster=w497, "integration time"=w498) -> (w496:T5)
          }
          frame "l" {
            w502 = u32 2 items=["short  ", "medium  ", "long  "] ("integration time 2")
            n143 = Bundle By Name(cluster=w501, "integration time"=w502, "Short/Long integration time"=w499) -> (w500:T5)
          }
        }
      }
      frame "pulsed" {
        n144 = Delete From Array(array=w515, index=0 ("Index")) -> (deleted portion=w516:string, array with subset deleted=w503:string[])  [unwired: 1 in]
        n145 = case shown="\"on\", Default" w516 {
          tunnel: w514 -> [w526 w529]
          tunnel: [w525 w528] -> w507
          tunnel: w503 -> [w523 _]
          frame "on", Default {
            w524 = u16 1 items=["Continuous", "Pulsed"] ("sweep method")
            n146 = Fract/Exp String To Number(string=w523) -> (number=w521:dbl[])  [unwired: 3 in, 1 out]
            n147 = Index Array(array=w521, index #1=0 ("Index")) -> (element #1=w520:dbl, element #2=w519:dbl, element #3=w518:dbl)  [unwired: 2 in]
            n148 = Bundle By Name(cluster=w526, "sweep method"=w524, "Pulse period"=w520, "Base voltage"=w519, "Pulse width"=w518) -> (w525:T5)
          }
          frame "off" {
            w527 = u16 0 items=["Continuous", "Pulsed"] ("sweep method")
            n149 = Bundle By Name(cluster=w529, "sweep method"=w527) -> (w528:T5)
          }
        }
      }
      frame "gaterangemode" {
        n150 = Delete From Array(array=w540, index=0 ("Index")) -> (deleted portion=w541:string)  [unwired: 1 in, 1 out]
        n151 = case shown="\"f\"" w541 {
          tunnel: [w543 w544 w545] -> w530
          frame "a", Default {
            w543 = u16 0 items=["Auto", "Limited", "Fixed"] ("Gate Range\nmode 2")
          }
          frame "f" {
            w544 = u16 2 items=["Auto", "Limited", "Fixed"] ("Gate Range\nmode 2")
          }
          frame "l" {
            w545 = u16 1 items=["Auto", "Limited", "Fixed"] ("Gate Range\nmode 2")
          }
        }
      }
      frame "gaterange" {
        (unwired) u8 11 items=["10fA  ", "100fA  ", "1nA  ", "10nA", "100nA", "1uA", "10uA", "100uA", "1mA", "10mA", "100mA", "1A"] ("Gate Range 2")
        n152 = Delete From Array(array=w563, index=0 ("Index")) -> (deleted portion=w553:string)  [unwired: 1 in, 1 out]
        n153 = Scan Value(string=w553, format string="") -> (value=w551:dbl)  [unwired: 1 in, 1 out]
        n154 = Logarithm Base 10(1:w551) -> (0:w550:dbl)
        n155 = Round To Nearest(number=w550) -> (nearest integer value=w549:dbl)
        n156 = Add(x=w549, y=11.0) -> (x+y=w547:dbl)
        n157 = To Unsigned Byte Integer(number=w547) -> (unsigned 8bit integer=w546:u8)
      }
      frame "drainrange" {
        (unwired) u8 11 items=["10fA  ", "100fA  ", "1nA  ", "10nA", "100nA", "1uA", "10uA", "100uA", "1mA", "10mA", "100mA", "1A"] ("Gate Range 2")
        n158 = Delete From Array(array=w582, index=0 ("Index")) -> (deleted portion=w573:string)  [unwired: 1 in, 1 out]
        n159 = Scan Value(string=w573, format string="") -> (value=w571:dbl)  [unwired: 1 in, 1 out]
        n160 = Logarithm Base 10(1:w571) -> (0:w570:dbl)
        n161 = Round To Nearest(number=w570) -> (nearest integer value=w569:dbl)
        n162 = Add(x=w569, y=11.0) -> (x+y=w567:dbl)
        n163 = To Unsigned Byte Integer(number=w567) -> (unsigned 8bit integer=w566:u8)
      }
      frame "drainrangemode" {
        n164 = Delete From Array(array=w594, index=0 ("Index")) -> (deleted portion=w595:string)  [unwired: 1 in, 1 out]
        n165 = case shown="\"f\"" w595 {
          tunnel: [w597 w598 w599] -> w584
          frame "a", Default {
            w597 = u16 0 items=["Auto", "Limited", "Fixed"] ("Gate Range\nmode 2")
          }
          frame "f" {
            w598 = u16 2 items=["Auto", "Limited", "Fixed"] ("Gate Range\nmode 2")
          }
          frame "l" {
            w599 = u16 1 items=["Auto", "Limited", "Fixed"] ("Gate Range\nmode 2")
          }
        }
      }
      frame "Error", Default {
      }
      frame "logfile" {
        n166 = Number To Decimal String(number=w640) -> (decimal integer string=w644:string)  [unwired: 1 in]
        n167 = Concatenate Strings(w642, "logfile" ("Substring"), w644, ".txt" ("Substring")) -> (w639:string)
        n168 = String To Path(string=w639) -> (path=w612:path)
        n169 = Unbundle(w638) -> ("integration time"=w637:u32, "Short/Long integration time"=w636:dbl, "hold time (sec)"=w635:dbl, "delay time (sec)"=w634:dbl, "Step Time (0 disables)"=w633:dbl, "sweep method"=w632:u16, "Pulse period"=w631:dbl, "Base voltage"=w630:dbl, "Pulse width"=w629:dbl)
        n170 = Build Array(w637, w636, w635, w634, w633, w632, w631, w630, w629, w623, w624, w625, w626, w627, w628) -> (w616:dbl[])
        n171 = Insert Into Array(array=dbl[][] [] ("Input Array"), new element=w616) -> (w615:dbl[][])  [unwired: 2 in]
        n172 = call <vilib>:"compatOverwrite.vi"("overwrite (F)"=TRUE) -> ("overwrite?"=w610:T7)
        n173 = Open/Create/Replace File(file path (use dialog)=w612, error in=w614, operation (0:open)=w610) -> (refnum out=w620:refnum<file>, error out=w619:errorcluster)  [unwired: 3 in, 1 out]
        n174 = call "4155C Write array to file.vi"("Byte Stream File Refnum"=w620, "Header"=string[] ["Int Time", "Short/Long Itime", "Hold time", "Delay time", "Step time", "Sweep method", "Pulse period", "Base Voltage", "Pulse width", "Drain compliance", "Gate compliance", "Gate range mode", "Gate range", "S/D range mode", "S/D range"], "Data Array"=w615, "error in (no error)"=w619) -> ("dup refnum"=w622:refnum<file>, "error out"=w621:errorcluster)  [unwired: 1 in]
        n175 = Close File(refnum=w622, error in=w621) -> (error out=w613:errorcluster)  [unwired: 1 out]
      }
      frame "sample" {
        n176 = Number To Decimal String(number=w693) -> (decimal integer string=w692:string)  [unwired: 1 in]
        n177 = Fract/Exp String To Number(string=w689) -> (number=w649:dbl[])  [unwired: 3 in, 1 out]
        n178 = Concatenate Strings(w667, "-sample-" ("Substring"), w692, ".txt" ("Substring")) -> (w690:string)
        n179 = String To Path(string=w690) -> (path=w671:path)
        n180 = Index Array(array=w649, index=0 ("Index")) -> (element=w687:dbl)
        n181 = Index Array(array=w649, index=2 ("Index")) -> (element=w683:dbl)
        n182 = Index Array(array=w649, index=3 ("Index")) -> (element=w652:dbl)
        n183 = Index Array(array=w649, index=4 ("Index")) -> (element=w648:dbl)
        n184 = call "4155C Config Sampling Measurements.vi"("Sampling interval"=w648, "Sample time"=w652, "Display on/off"=TRUE, "Timings"=w658, "Num Points"=w683, "error in (no error)"=w695, "Drain Compliance"=w694, "Gate Compliance"=w668, "VISA session"=w696) -> ("error out"=w697:errorcluster, "dup VISA resource name"=w698:refnum<visa-resource-name>)  [unwired: 1 in]
        n185 = Index Array(array=w649, index=1 ("Index")) -> (element=w684:dbl)
        n186 = call "4155C Take Sample.vi"("Emergency Stop"=w664, "error in (no error)"=w697, "Vd"=w684, "Vg"=w687, "VISA resource name in"=w698) -> ("error out"=w662:errorcluster, "Id"=w700:dbl[], "Ig"=w673:dbl[], "VISA Resource Name out"=w660:refnum<visa-resource-name>, "Is"=w699:dbl[], "Time"=w677:dbl[])  [unwired: 1 in]
        n187 = Insert Into Array(array=dbl[][] [] ("Input Array"), new element=w677) -> (w676:dbl[][])  [unwired: 2 in]
        n188 = Insert Into Array(array=w676, new element=w673) -> (w675:dbl[][])  [unwired: 2 in]
        n189 = Insert Into Array(array=w675, new element=w700) -> (w674:dbl[][])  [unwired: 2 in]
        n190 = VISA Write(VISA resource name=w660, write buffer=":DISP ON" ("write buffer (\"\")"), error in (no error)=w662) -> (VISA resource name out=w659:refnum<visa-resource-name>, error out=w661:errorcluster)  [unwired: 1 out]
        n191 = Insert Into Array(array=w674, new element=w699) -> (w666:dbl[][])  [unwired: 2 in]
        n192 = Transpose 2D Array(2D array=w666) -> (transposed array=w665:dbl[][])
        n193 = call <vilib>:"compatOverwrite.vi"("overwrite (F)"=TRUE) -> ("overwrite?"=w646:T7)
        n194 = Open/Create/Replace File(file path (use dialog)=w671, error in=w661, operation (0:open)=w646) -> (refnum out=w680:refnum<file>, error out=w679:errorcluster)  [unwired: 3 in, 1 out]
        n195 = call "4155C Write array to file.vi"("Byte Stream File Refnum"=w680, "Header"=string[] ["Time /s", "Ig /A", "Id /A", "Is /A"], "Data Array"=w665, "error in (no error)"=w679) -> ("dup refnum"=w682:refnum<file>, "error out"=w681:errorcluster)  [unwired: 1 in]
        n196 = Close File(refnum=w682, error in=w681) -> (error out=w669:errorcluster)  [unwired: 1 out]
      }
      frame "samplei" {
        n197 = Number To Decimal String(number=w751) -> (decimal integer string=w750:string)  [unwired: 1 in]
        n198 = Fract/Exp String To Number(string=w747) -> (number=w713:dbl[])  [unwired: 3 in, 1 out]
        n199 = Concatenate Strings(w729, "-samplei-" ("Substring"), w750, ".txt" ("Substring")) -> (w748:string)
        n200 = String To Path(string=w748) -> (path=w732:path)
        n201 = Index Array(array=w713, index=4 ("Index")) -> (element=w707:dbl)
        n202 = Index Array(array=w713, index=3 ("Index")) -> (element=w708:dbl)
        n203 = Index Array(array=w713, index=1 ("Index")) -> (element=w710:dbl)
        n204 = Index Array(array=w713, index=0 ("Index")) -> (element=w711:dbl)
        n205 = Index Array(array=w713, index=2 ("Index")) -> (element=w709:dbl)
        n206 = call "4155C Config SamplingI Measurements.vi"("Sample time"=w709, "Display on/off"=TRUE, "Timings"=w721, "Num Points"=w710, "error in (no error)"=w753, "Sampling interval"=w708, "VISA session"=w754) -> ("error out"=w755:errorcluster, "dup VISA resource name"=w756:refnum<visa-resource-name>)  [unwired: 3 in]
        n207 = call "4155C Take SampleI.vi"("Emergency Stop"=w726, "error in (no error)"=w755, "Idg 2"=w711, "Vdg compliance 2"=w707, "VISA resource name in"=w756) -> ("error out"=w724:errorcluster, "Idg"=w758:dbl[], "Vdg"=w734:dbl[], "VISA Resource Name out"=w722:refnum<visa-resource-name>, "Is"=w757:dbl[], "Time"=w738:dbl[])  [unwired: 1 in]
        n208 = Insert Into Array(array=dbl[][] [] ("Input Array"), new element=w738) -> (w737:dbl[][])  [unwired: 2 in]
        n209 = Insert Into Array(array=w737, new element=w734) -> (w736:dbl[][])  [unwired: 2 in]
        n210 = Insert Into Array(array=w736, new element=w758) -> (w735:dbl[][])  [unwired: 2 in]
        n211 = VISA Write(VISA resource name=w722, write buffer=":DISP ON" ("write buffer (\"\")"), error in (no error)=w724) -> (VISA resource name out=w706:refnum<visa-resource-name>, error out=w723:errorcluster)  [unwired: 1 out]
        n212 = Insert Into Array(array=w735, new element=w757) -> (w728:dbl[][])  [unwired: 2 in]
        n213 = Transpose 2D Array(2D array=w728) -> (transposed array=w727:dbl[][])
        n214 = call <vilib>:"compatOverwrite.vi"("overwrite (F)"=TRUE) -> ("overwrite?"=w701:T7)
        n215 = Open/Create/Replace File(file path (use dialog)=w732, error in=w723, operation (0:open)=w701) -> (refnum out=w741:refnum<file>, error out=w740:errorcluster)  [unwired: 3 in, 1 out]
        n216 = call "4155C Write array to file.vi"("Byte Stream File Refnum"=w741, "Header"=string[] ["Time /s", "Vdg /V", "Idg /A", "Is /A"], "Data Array"=w727, "error in (no error)"=w740) -> ("dup refnum"=w743:refnum<file>, "error out"=w742:errorcluster)  [unwired: 1 in]
        n217 = Close File(refnum=w743, error in=w742) -> (error out=w704:errorcluster)  [unwired: 1 out]
        n218 = VISA Write(VISA resource name=w706, write buffer=";:PAGE:SCON:STAN OFF;:PAGE:CHAN:VSU2:DIS;" ("write buffer (\"\")"), error in (no error)=w704) -> (VISA resource name out=w702:refnum<visa-resource-name>, error out=w703:errorcluster)  [unwired: 1 out]
      }
      frame "#" {
        n219 = VISA Write(VISA resource name=w763, write buffer=":DISP ON" ("write buffer (\"\")"), error in (no error)=w762) -> (VISA resource name out=w761:refnum<visa-resource-name>, error out=w760:errorcluster)  [unwired: 1 out]
      }
      frame "stressV" {
        n220 = Number To Decimal String(number=w811) -> (decimal integer string=w810:string)  [unwired: 1 in]
        n221 = Fract/Exp String To Number(string=w807) -> (number=w779:dbl[])  [unwired: 3 in, 1 out]
        n222 = Concatenate Strings(w794, "-stressV-" ("Substring"), w810, ".txt" ("Substring")) -> (w808:string)
        n223 = String To Path(string=w808) -> (path=w798:path)
        n224 = Index Array(array=w779, index=3 ("Index")) -> (element=w776:dbl)
        n225 = Index Array(array=w779, index=1 ("Index")) -> (element=w774:dbl)
        n226 = Index Array(array=w779, index=0 ("Index")) -> (element=w773:dbl)
        n227 = Index Array(array=w779, index=4 ("Index")) -> (element=w778:dbl)
        n228 = Index Array(array=w779, index=2 ("Index")) -> (element=w775:dbl)
        n229 = call "4155C Config V Stress.vi"("VISA session"=w814, "ID compliance"=w776, "VD"=w774, "VG"=w773, "IG compliance"=w775, "error in (no error)"=w813, "Display on/off"=TRUE) -> ("dup VISA resource name"=w816:refnum<visa-resource-name>, "error out"=w815:errorcluster)
        n230 = call "4155C Apply Stress.vi"("error in (no error)"=w815, "Duration"=w778, "Emergency Stop"=w793, "VISA resource name in"=w816) -> ("error out"=w791:errorcluster, "VISA Resource Name out"=w789:refnum<visa-resource-name>)
        n231 = VISA Write(VISA resource name=w789, write buffer=":DISP ON" ("write buffer (\"\")"), error in (no error)=w791) -> (VISA resource name out=w788:refnum<visa-resource-name>, error out=w790:errorcluster)  [unwired: 1 out]
        n232 = call <vilib>:"compatOverwrite.vi"("overwrite (F)"=TRUE) -> ("overwrite?"=w772:T7)
        n233 = Open/Create/Replace File(file path (use dialog)=w798, error in=w790, operation (0:open)=w772) -> (refnum out=w801:refnum<file>, error out=w800:errorcluster)  [unwired: 3 in, 1 out]
        n234 = call "4155C Write array to file.vi"("Byte Stream File Refnum"=w801, "Header"=string[] ["V stress completed successfully", ""], "error in (no error)"=w800) -> ("dup refnum"=w803:refnum<file>, "error out"=w802:errorcluster)  [unwired: 2 in]
        n235 = Close File(refnum=w803, error in=w802) -> (error out=w796:errorcluster)  [unwired: 1 out]
      }
      frame "stressI" {
        n236 = Number To Decimal String(number=w852) -> (decimal integer string=w851:string)  [unwired: 1 in]
        n237 = Fract/Exp String To Number(string=w848) -> (number=w822:dbl[])  [unwired: 3 in, 1 out]
        n238 = Concatenate Strings(w835, "-stressI-" ("Substring"), w851, ".txt" ("Substring")) -> (w849:string)
        n239 = String To Path(string=w849) -> (path=w839:path)
        n240 = Index Array(array=w822, index=1 ("Index")) -> (element=w818:dbl)
        n241 = Index Array(array=w822, index=0 ("Index")) -> (element=w819:dbl)
        n242 = call "4155C Config I Stress.vi"("VISA session"=w855, "IDG"=w819, "VDG compliance"=w818, "error in (no error)"=w854, "Display on/off"=TRUE) -> ("dup VISA resource name"=w857:refnum<visa-resource-name>, "error out"=w856:errorcluster)
        n243 = Index Array(array=w822, index=2 ("Index")) -> (element=w820:dbl)
        n244 = call "4155C Apply Stress.vi"("error in (no error)"=w856, "Duration"=w820, "Emergency Stop"=w834, "VISA resource name in"=w857) -> ("error out"=w832:errorcluster, "VISA Resource Name out"=w830:refnum<visa-resource-name>)
        n245 = VISA Write(VISA resource name=w830, write buffer=":DISP ON" ("write buffer (\"\")"), error in (no error)=w832) -> (VISA resource name out=w829:refnum<visa-resource-name>, error out=w831:errorcluster)  [unwired: 1 out]
        n246 = call <vilib>:"compatOverwrite.vi"("overwrite (F)"=TRUE) -> ("overwrite?"=w817:T7)
        n247 = Open/Create/Replace File(file path (use dialog)=w839, error in=w831, operation (0:open)=w817) -> (refnum out=w842:refnum<file>, error out=w841:errorcluster)  [unwired: 3 in, 1 out]
        n248 = call "4155C Write array to file.vi"("Byte Stream File Refnum"=w842, "Header"=string[] ["I stress completed successfully", ""], "error in (no error)"=w841) -> ("dup refnum"=w844:refnum<file>, "error out"=w843:errorcluster)  [unwired: 2 in]
        n249 = Close File(refnum=w844, error in=w843) -> (error out=w837:errorcluster)  [unwired: 1 out]
      }
      frame "vsu2pulse" {
        n250 = Number To Decimal String(number=w891) -> (decimal integer string=w890:string)  [unwired: 1 in]
        n251 = Fract/Exp String To Number(string=w887) -> (number=w862:dbl[])  [unwired: 3 in, 1 out]
        n252 = Concatenate Strings(w875, "-vsu2-" ("Substring"), w890, ".txt" ("Substring")) -> (w888:string)
        n253 = String To Path(string=w888) -> (path=w879:path)
        n254 = Index Array(array=w862, index=1 ("Index")) -> (element=w861:dbl)
        n255 = Index Array(array=w862, index=0 ("Index")) -> (element=w859:dbl)
        n256 = call "4155C Config VSU2 Stress.vi"("error in (no error)"=w893, "VSU2"=w859, "Display on/off"=TRUE, "VISA session"=w894) -> ("error out"=w895:errorcluster, "dup VISA resource name"=w896:refnum<visa-resource-name>)
        n257 = call "4155C Apply Stress.vi"("error in (no error)"=w895, "Duration"=w861, "Emergency Stop"=w874, "VISA resource name in"=w896) -> ("error out"=w872:errorcluster, "VISA Resource Name out"=w870:refnum<visa-resource-name>)
        n258 = VISA Write(VISA resource name=w870, write buffer=":DISP ON" ("write buffer (\"\")"), error in (no error)=w872) -> (VISA resource name out=w869:refnum<visa-resource-name>, error out=w871:errorcluster)  [unwired: 1 out]
        n259 = call <vilib>:"compatOverwrite.vi"("overwrite (F)"=TRUE) -> ("overwrite?"=w858:T7)
        n260 = Open/Create/Replace File(file path (use dialog)=w879, error in=w871, operation (0:open)=w858) -> (refnum out=w882:refnum<file>, error out=w881:errorcluster)  [unwired: 3 in, 1 out]
        n261 = call "4155C Write array to file.vi"("Byte Stream File Refnum"=w882, "Header"=string[] ["VSU2 pulse completed successfully", ""], "error in (no error)"=w881) -> ("dup refnum"=w884:refnum<file>, "error out"=w883:errorcluster)  [unwired: 2 in]
        n262 = Close File(refnum=w884, error in=w883) -> (error out=w877:errorcluster)  [unwired: 1 out]
      }
      frame "sample-fpp" {
        w904 = string[] ["Time /s", "Id VgVd /A", "Ig VgVd /A", "Vp1 VgVd /V", "Vp2 VgVd /V"] ("Header")
        w908 = "%d" ("format string")
        n263 = Number To Decimal String(number=w958) -> (decimal integer string=w957:string)  [unwired: 1 in]
        n264 = Fract/Exp String To Number(string=w954) -> (number=w942:dbl[])  [unwired: 3 in, 1 out]
        n265 = Concatenate Strings(w948, "-samplefpp-" ("Substring"), w957, ".txt" ("Substring")) -> (w955:string)
        n266 = String To Path(string=w955) -> (path=w916:path)
        n267 = Index Array(array=w942, index=0 ("Index")) -> (element=w902:dbl)
        n268 = Index Array(array=w942, index=1 ("Index")) -> (element=w901:dbl)
        n269 = Index Array(array=w942, index=2 ("Index")) -> (element=w950:dbl)
        n270 = Index Array(array=w942, index=3 ("Index")) -> (element=w940:dbl)
        n271 = call "4155C Config Sampling Measurements FPP.vi"("VISA session"=w961, "Num Points"=w950, "Vg"=w902, "Display on/off"=TRUE, "Gate Compliance"=w949, "Drain Compliance"=w959, "Standby"="Standby", "error in (no error)"=w960, "Timings"=w947, "Vd"=w901, "Sample time"=w940) -> ("dup VISA resource name"=w918:refnum<visa-resource-name>, "error out"=w917:errorcluster)  [unwired: 3 in]
        n272 = Number To Decimal String(number=w902) -> (decimal integer string=w928:string)  [unwired: 1 in]
        n273 = call "4155C Take Sample FPP.vi"("VISA resource name in"=w918, "error in (no error)"=w917, "Emergency Stop"=w919) -> ("Time"=w923:dbl[], "Vp1"=w933:dbl[], "VISA Resource Name out"=w899:refnum<visa-resource-name>, "Ig"=w921:dbl[], "Id"=w922:dbl[], "Vp2"=w931:dbl[], "error out"=w920:errorcluster)  [unwired: 10 in]
        n274 = Insert Into Array(array=dbl[][] [] ("Input Array"), new element=w923) -> (w937:dbl[][])  [unwired: 2 in]
        n275 = Number To Decimal String(number=w901) -> (decimal integer string=w926:string)  [unwired: 1 in]
        n276 = Insert Into Array(array=w937, new element=w922) -> (w936:dbl[][])  [unwired: 2 in]
        n277 = Concatenate Strings("(Vg = " ("Substring"), w928, "V, Vd = " ("Substring"), w926, "V)" ("Substring")) -> (w924:string)
        n278 = Insert Into Array(array=w936, new element=w921) -> (w935:dbl[][])  [unwired: 2 in]
        n279 = Insert Into Array(array=w935, new element=w933) -> (w932:dbl[][])  [unwired: 2 in]
        n280 = Insert Into Array(array=w932, new element=w931) -> (w900:dbl[][])  [unwired: 2 in]
        n281 = call <vilib>:"compatOverwrite.vi"("overwrite (F)"=TRUE) -> ("overwrite?"=w897:T7)
        n282 = Open/Create/Replace File(file path (use dialog)=w916, error in=w920, operation (0:open)=w897) -> (refnum out=w913:refnum<file>, error out=w914:errorcluster)  [unwired: 3 in, 1 out]
        n283 = Array To Spreadsheet String(array=w904, 3:w908) -> (spreadsheet string=w910:string)  [unwired: 1 in]
        n284 = Transpose 2D Array(2D array=w900) -> (transposed array=w930:dbl[][])
        n285 = Search and Replace String(replace all?=TRUE ("replace all? (F)"), input string=w910, search string="VgVd", replace string=w924) -> (result string=w906:string)  [unwired: 4 in, 3 out]
        n286 = Spreadsheet String To Array(format string=w908, spreadsheet string=w906, array type (2D Dbl)=w904) -> (array=w905:string[])  [unwired: 1 in]
        n287 = call "4155C Write array to file.vi"("Byte Stream File Refnum"=w913, "Header"=w905, "Data Array"=w930, "error in (no error)"=w914) -> ("dup refnum"=w911:refnum<file>, "error out"=w912:errorcluster)  [unwired: 1 in]
        n288 = Close File(refnum=w911, error in=w912) -> (error out=w898:errorcluster)  [unwired: 1 out]
      }
      frame "resample-fpp" {
        w971 = string[] ["Time /s", "Id VgVd /A", "Ig VgVd /A", "Vp1 VgVd /V", "Vp2 VgVd /V"] ("Header")
        w975 = "%d" ("format string")
        n289 = Number To Decimal String(number=w1017) -> (decimal integer string=w1016:string)  [unwired: 1 in]
        n290 = Fract/Exp String To Number(string=w1013) -> (number=w964:dbl[])  [unwired: 3 in, 1 out]
        n291 = Concatenate Strings(w1009, "-resamplefpp-" ("Substring"), w1016, ".txt" ("Substring")) -> (w1014:string)
        n292 = String To Path(string=w1014) -> (path=w983:path)
        n293 = Index Array(array=w964, index=0 ("Index")) -> (element=w970:dbl)
        n294 = Index Array(array=w964, index=1 ("Index")) -> (element=w969:dbl)
        n295 = Number To Decimal String(number=w970) -> (decimal integer string=w993:string)  [unwired: 1 in]
        n296 = call "4155C Take Sample FPP.vi"("VISA resource name in"=w966, "error in (no error)"=w965, "Emergency Stop"=w984) -> ("Time"=w988:dbl[], "Vp1"=w998:dbl[], "VISA Resource Name out"=w968:refnum<visa-resource-name>, "Ig"=w986:dbl[], "Id"=w987:dbl[], "Vp2"=w996:dbl[], "error out"=w985:errorcluster)  [unwired: 10 in]
        n297 = Insert Into Array(array=dbl[][] [] ("Input Array"), new element=w988) -> (w1002:dbl[][])  [unwired: 2 in]
        n298 = Number To Decimal String(number=w969) -> (decimal integer string=w991:string)  [unwired: 1 in]
        n299 = Insert Into Array(array=w1002, new element=w987) -> (w1001:dbl[][])  [unwired: 2 in]
        n300 = Concatenate Strings("(Vg = " ("Substring"), w993, "V, Vd = " ("Substring"), w991, "V)" ("Substring")) -> (w989:string)
        n301 = Insert Into Array(array=w1001, new element=w986) -> (w1000:dbl[][])  [unwired: 2 in]
        n302 = Insert Into Array(array=w1000, new element=w998) -> (w997:dbl[][])  [unwired: 2 in]
        n303 = Insert Into Array(array=w997, new element=w996) -> (w963:dbl[][])  [unwired: 2 in]
        n304 = call <vilib>:"compatOverwrite.vi"("overwrite (F)"=TRUE) -> ("overwrite?"=w962:T7)
        n305 = Open/Create/Replace File(file path (use dialog)=w983, error in=w985, operation (0:open)=w962) -> (refnum out=w980:refnum<file>, error out=w981:errorcluster)  [unwired: 3 in, 1 out]
        n306 = Array To Spreadsheet String(array=w971, 3:w975) -> (spreadsheet string=w977:string)  [unwired: 1 in]
        n307 = Transpose 2D Array(2D array=w963) -> (transposed array=w995:dbl[][])
        n308 = Search and Replace String(replace all?=TRUE ("replace all? (F)"), input string=w977, search string="VgVd", replace string=w989) -> (result string=w973:string)  [unwired: 4 in, 3 out]
        n309 = Spreadsheet String To Array(format string=w975, spreadsheet string=w973, array type (2D Dbl)=w971) -> (array=w972:string[])  [unwired: 1 in]
        n310 = call "4155C Write array to file.vi"("Byte Stream File Refnum"=w980, "Header"=w972, "Data Array"=w995, "error in (no error)"=w981) -> ("dup refnum"=w978:refnum<file>, "error out"=w979:errorcluster)  [unwired: 1 in]
        n311 = Close File(refnum=w978, error in=w979) -> (error out=w967:errorcluster)  [unwired: 1 out]
      }
    }
    n312 = local write "Lines left to run:"(w39) -> ()
    n313 = Empty String/Path?(string/path=w39) -> (empty?=w75:bool)
    n314 = Not(x=w75) -> (.not. x?=w74:bool)
  }
